vi "Error Converter(ErrCheck).vi"(8 "error in (no error)":errorcluster) -> (0 "error out":errorcluster)   [LabVIEW 2026, in "MrcLib.lvlib"]
uses:
  <userlib>/MRC/MrcLib/MrcLib.lvlib
panel:
  in  "string":string="This error is returned by the shared library function."
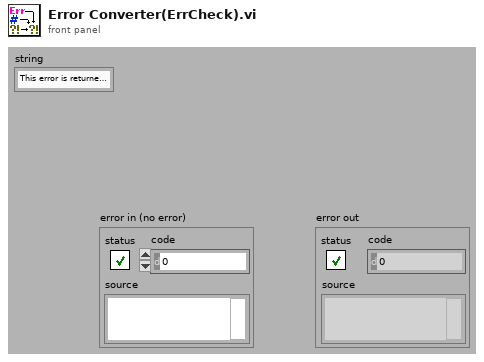
[diagram p1: front panel]
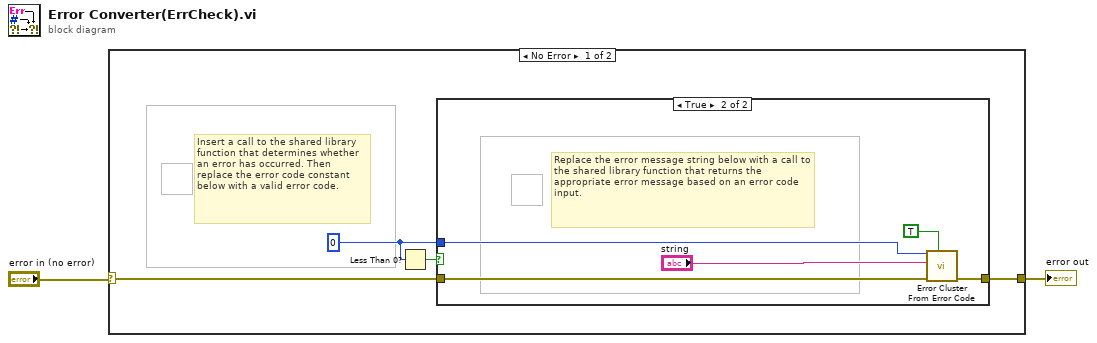
[diagram p0: block diagram]
diagram:
  n1 = case shown="No Error" "error in (no error)" {
    selector: "error in (no error)" -> [w5 w13]
    tunnel: [w4 w13] -> w1
    frame No Error {
      w3 = 0 ("Error Code")
      # "Insert a call to the shared library function that determines whether an error has occurred. Then replace the error code constant below with a valid error code."
      n2 = Less Than 0?(x=w3) -> (x < 0?=w6:bool)
      n3 = case shown="True" w6 {
        tunnel: w5 -> [w7 w9]
        tunnel: w3 -> [_ w11]
        tunnel: [w7 w8] -> w4
        frame False {
        }
        frame True {
          # "Replace the error message string below with a call to the shared library function that returns the appropriate error message based on an error code input."
          n4 = call <vilib>:"Error Cluster From Error Code.vi"("show call chain? (False)"=TRUE, "error in (no error)"=w9, "error message (\"\")"="string", "error code (0)"=w11) -> ("error out"=w8:errorcluster)  [unwired: 5 in]
        }
      }
    }
    frame Error {
    }
  }
  "error out" <- w1
